vi "Proccess Async Lockin Channel.vi"(4 "Lock-in settings":T1={"Averaging period, s"=0.0, "Output Representation"=enum."Real/Imaginary", "Output value"=enum."RMS", "Phase delay, points"=0} {"Averaging period, s" format="%#_6p"}, 5 "Channel info":T2, 6 "Overwrite\nclock, Hz":dbl, 7 "Raw chunk size":i64, 8 "error in (no error)":errorcluster, 9 "Settings":string, 10 "group name":string, 11 "Data file path":path) -> (0 "error out":errorcluster, 1 "Settings out":string, 2 "Channel Length":u64, 3 "signal(s) out":waveform(dbl)[](array[waveform]))   [LabVIEW 2016]
uses:
  CH_name_pts_phase.ctl
  Syncronous Lockin Settings.ctl
  Utilities/Replace dt SGL.vi
  <vilib>/Waveform/WDTOps.llb/WDT Append Waveforms DBL.vi
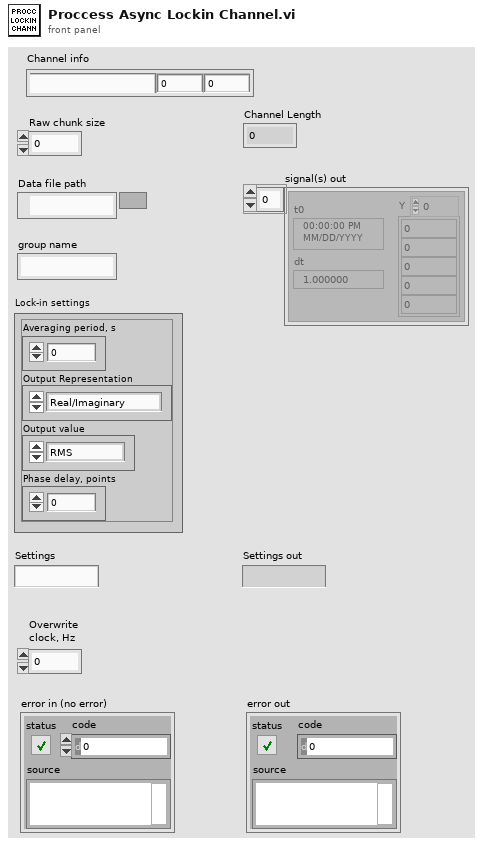
[diagram p1: front panel]
types:
  T1 = typedef "Syncronous Lockin Settings.ctl" = cluster{"Averaging period, s":dbl, "Output Representation":enum16{"Real/Imaginary", "Polar"}, "Output value":enum16{"Amplitude", "RMS", "Peak-to-Peak"}, "Phase delay, points":i32}
  T2 = typedef "CH_name_pts_phase.ctl" = cluster{"Channel":string, "pts per sine wave":i32, "Phase":dbl}
  T3 = enum16{"open", "open or create", "create or replace", "create", "open (read-only)"}
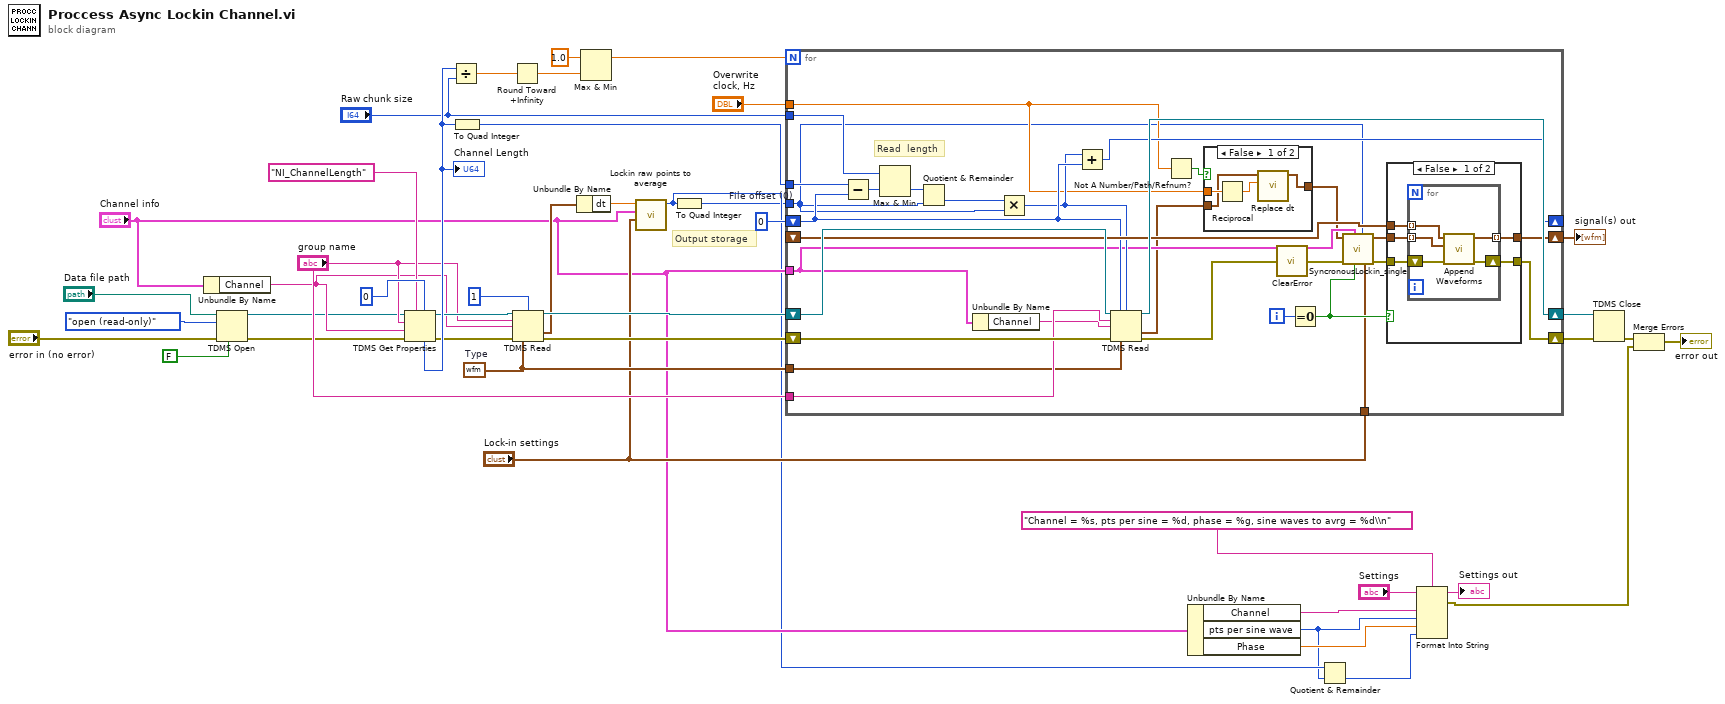
[diagram p0: block diagram]
diagram:
  w21 = waveform(sgl) {"t0"=timestamp(0 s since 1904-01-01), "dt"=1.0, "Y"=[]}  # Type
  w33 = i64 0  # File offset (0)
  # "Output storage"
  n1 = Unbundle By Name("Channel info") -> ("Channel"=w22:string)
  n2 = TDMS Open(6:FALSE ("disable buffering (T)"), 8:"error in (no error)", 10:T3."open (read-only)" ("TDMS open mode"), 11:"Data file path") -> (0:w2:errorcluster, 3:w3:refnum<k34>)  [unwired: 3 in]
  n3 = TDMS Get Properties(5:u64 0, 7:"NI_ChannelLength" ("property name"), 8:w2, 9:w22, 10:"group name", 11:w3) -> (0:w27:errorcluster, 3:w25:refnum<k34>, 4:w39:u64)  [unwired: 3 out]
  "Channel Length" <- w39
  n4 = Divide(x=w39, y="Raw chunk size") -> (x/y=w31:dbl)
  n5 = To Quad Integer(1:w39) -> (0:w40:i64)
  n6 = Round Toward +Infinity(x=w31) -> (ceil(x): smallest int >= x=w32:dbl)
  n7 = TDMS Read(0:w25, 2:i64 1 ("count (-1: all)"), 5:"group name", 7:w22, 11:w27, 12:w21) -> (4:w24:refnum<k34>, 10:w19:waveform(sgl), 15:w26:errorcluster)  [unwired: 2 in, 3 out]
  n8 = Unbundle By Name(w19) -> ("dt"=w18:dbl)
  n9 = Max & Min(x=1.0, y=w32) -> (max(x,y)=w37:dbl)  [unwired: 1 out]
  n10 = call "Lockin raw points to average.vi"("Lock-in settings"="Lock-in settings", "CH name                          points   phase"="Channel info", "dt"=w18) -> ("Lockin raw points to average"=w5:i32)  [unwired: 8 in]
  n11 = To Quad Integer(1:w5) -> (0:w1:i64)
  n12 = for {
    N: w37 -> [_]
    shift-right: [w61] -> w16
    shift-left: w26 -> [w74]
    shift-right: [w71] -> w35
    shift-left: w24 -> [w73]
    tunnel: "group name" -> [w72]
    tunnel: "Channel info" -> [w50]
    shift-right: [w70] -> _
    shift-left: w33 -> [w60]
    tunnel: "Raw chunk size" -> [w54]
    tunnel: w21 -> [w69]
    shift-right: [w66] -> w43
    shift-left: _ -> [w65]
    tunnel: w1 -> [w46]
    tunnel: w40 -> [w55]
    tunnel: "Overwrite\nclock, Hz" -> [w53]
    tunnel: "Lock-in settings" -> [w45]
    i -> [w67]
    # "Read  length"
    n13 = Subtract(x=w55, y=w60) -> (x-y=w59:i64)
    n14 = Max & Min(x=w54, y=w59) -> (min(x,y)=w58:i64)  [unwired: 1 out]
    n15 = Quotient & Remainder(x=w58, y=w46) -> (floor(x/y)=w57:i64)  [unwired: 1 out]
    n16 = Unbundle By Name(w50) -> ("Channel"=w51:string)
    n17 = Multiply(x=w57, y=w46) -> (x*y=w56:i64)
    n18 = Add(x=w56, y=w60) -> (x+y=w70:i64)
    n19 = TDMS Read(0:w73, 1:w60, 2:w56, 5:w72, 7:w51, 11:w74, 12:w69) -> (4:w71:refnum<k34>, 10:w48:waveform(sgl), 15:w52:errorcluster)  [unwired: 1 in, 3 out]
    n20 = Not A Number/Path/Refnum?(number/path/refnum=w53) -> (NaN/Path/Refnum?=w49:bool)
    n21 = case shown="False" w49 {
      tunnel: w48 -> [w76 w79]
      tunnel: [w78 w79] -> w47
      tunnel: w53 -> [w77 _]
      frame False {
        n22 = Reciprocal(x=w77) -> (1/x=w75:dbl)
        n23 = call-poly "Replace dt.vi"("dt"=w75, "Waveform in"=w76) -> ("Waveform out"=w78:waveform(sgl))  [unwired: 9 in]
      }
      frame True {
      }
    }
    n24 = call <vilib>:"ClearError.vi"("error in (no error)"=w52) -> ("error out"=w68:errorcluster)
    n25 = Equal To 0?(x=w67) -> (x = 0?=w64:bool)
    n26 = call "SyncronousLockin_single.vi"("Lock-in settings"=w45, "Raw points to average"=w46, "First chunk?"=w64, "CH name                          points   phase"=w50, "error in (no error)"=w68, "Data"=w47) -> ("error out"=w63:errorcluster, "signal(s) out"=w62:waveform(dbl)[])  [unwired: 4 in]
    n27 = case shown="False" w64 {
      tunnel: [w84 w91] -> w66
      tunnel: w65 -> [w82 _]
      tunnel: w63 -> [w83 w90]
      tunnel: w62 -> [w81 w91]
      tunnel: [w80 w90] -> w61
      frame False {
        n28 = for {
          tunnel: [w89] -> w84 mode=indexing
          tunnel: w82 -> [w88] mode=indexing
          shift-right: [w86] -> w80
          shift-left: w83 -> [w87]
          tunnel: w81 -> [w85] mode=indexing
          n29 = call-poly <vilib>:"Append Waveforms.vi"("error in (no error)"=w87, "waveform B"=w85, "waveform A"=w88) -> ("error out"=w86:errorcluster, "waveform out"=w89:waveform(dbl))  [unwired: 7 out]
        }
      }
      frame True {
      }
    }
  }
  "signal(s) out" <- w43
  n30 = Unbundle By Name("Channel info") -> ("Channel"=w12:string, "pts per sine wave"=w4:i32, "Phase"=w11:dbl)
  n31 = Quotient & Remainder(x=w5, y=w4) -> (floor(x/y)=w6:i32)  [unwired: 1 out]
  n32 = Format Into String(format string="Channel = %s, pts per sine = %d, phase = %g, sine waves to avrg = %d\\n", initial string="Settings", w12, w4, w11, w6) -> (resulting string=→"Settings out":string, error out=w7:errorcluster)  [unwired: 1 in]
  n33 = TDMS Close(8:w16, 11:w35) -> (0:w15:errorcluster)  [unwired: 1 out]
  n34 = Merge Errors(w15, w7) -> (→"error out":errorcluster)
